vi "LookAheadPoint.vi"(8 "Robot":cluster{"x":dbl, "y":dbl}, 9 "Spacing":dbl, 10 "LookAhead":dbl, 11 "Path":cluster{"x":dbl, "y":dbl}[](array[cluster])) -> (3 "Point":cluster{"x":dbl, "y":dbl})   [LabVIEW 2016]
panel:
  out "Index":i32
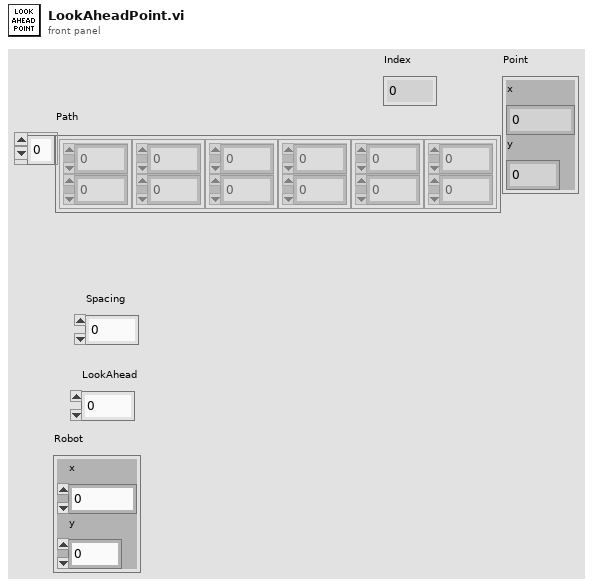
[diagram p1: front panel]
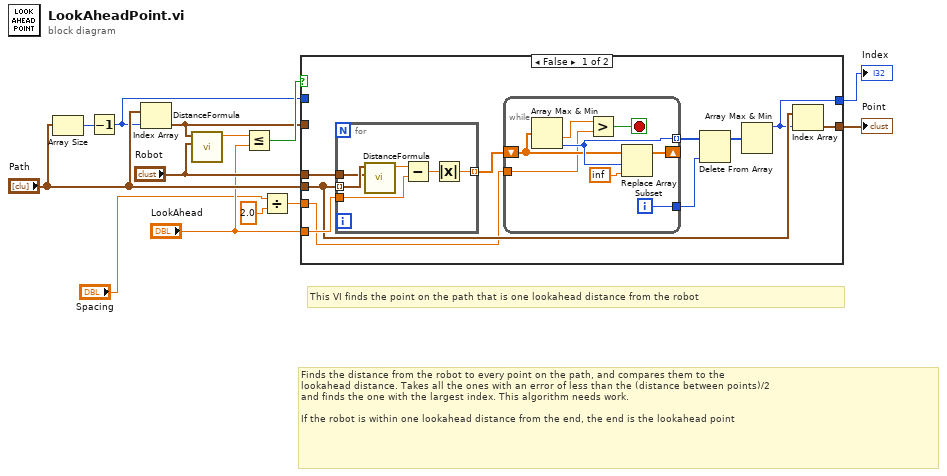
[diagram p0: block diagram]
diagram:
  # "This VI finds the point on the path that is one lookahead distance from the robot"
  # "Finds the distance from the robot to every point on the path, and compares them to the\nlookahead distance. Takes all the ones with an error of less than the (distance between points)/2\nand finds the one with the largest index. This algorithm needs work.\n\nIf the robot is within one lookahead distance from the end, the end is the lookahead point"
  n1 = Array Size(array="Path") -> (size(s)=w11:i32)
  n2 = Decrement(x=w11) -> (x-1=w5:i32)
  n3 = Index Array(array="Path", index=w5) -> (element=w6:cluster{"x":dbl, "y":dbl})
  n4 = call "DistanceFormula.vi"("Point 2"="Robot", "Point 1"=w6) -> ("Distance"=w8:dbl)  [unwired: 9 in]
  n5 = Less Or Equal?(x=w8, y="LookAhead") -> (x <= y?=w7:bool)
  n6 = Divide(x="Spacing", y=2.0) -> (x/y=w2:dbl)
  n7 = case shown="False" w7 {
    tunnel: "LookAhead" -> [w23 _]
    tunnel: [w22 w39] -> w13
    tunnel: "Path" -> [w21 _]
    tunnel: "Robot" -> [w20 _]
    tunnel: [w18 w38] -> w12
    tunnel: w6 -> [_ w39]
    tunnel: w5 -> [_ w38]
    tunnel: w2 -> [w17 _]
    frame False {
      n8 = for {
        tunnel: w21 -> [w37] mode=indexing
        tunnel: w20 -> [w36]
        tunnel: w23 -> [w34]
        tunnel: [w32] -> w19 mode=indexing
        n9 = call "DistanceFormula.vi"("Point 2"=w36, "Point 1"=w37) -> ("Distance"=w35:dbl)  [unwired: 9 in]
        n10 = Subtract(x=w35, y=w34) -> (x-y=w33:dbl)
        n11 = Absolute Value(x=w33) -> (abs(x)=w32:dbl)
      }
      n12 = while {
        tunnel: [w31] -> w16 mode=indexing
        shift-right: [w28] -> _
        shift-left: w19 -> [w29]
        tunnel: w17 -> [w26]
        tunnel: [w24] -> w15
        i -> [w24]
        stop <- w25 stop-if-true
        n13 = Array Max & Min(array=w29) -> (min value=w27:dbl, min index (indices)=w31:i32)  [unwired: 2 out]
        n14 = Greater?(x=w27, y=w26) -> (0:w25:bool)
        n15 = Replace Array Subset(array=w29, new element=inf, index=w31) -> (w28:dbl[])
      }
      n16 = Delete From Array(array=w16, index=w15) -> (array with subset deleted=w14:i32[])  [unwired: 1 in, 1 out]
      n17 = Array Max & Min(array=w14) -> (max value=w18:i32)  [unwired: 3 out]
      n18 = Index Array(array=w21, index=w18) -> (element=w22:cluster{"x":dbl, "y":dbl})
    }
    frame True {
    }
  }
  "Point" <- w13
  "Index" <- w12
